vi "Load SA Parametersvi.vi"(8 "error in (no error)":errorcluster, 11 "Skyworks Spur Test in":refnum<class "Skyworks Spur Test.lvclass">) -> (0 "error out":errorcluster, 3 "Skyworks Spur Test out":refnum<class "Skyworks Spur Test.lvclass">)   [LabVIEW 2018, in "Skyworks Spur Test.lvlib" / "Skyworks Spur Test.lvclass"]
uses:
  Skyworks Spur Test.lvclass
  C:/Sequence Automation/Plugins/Measurement Interface.lvlibp/Measurement Interface.lvclass
  Controls/SA Parameters.ctl
  Skyworks Spur Test.lvclass/Skyworks Spur Test.ctl
  Write SA Parameters.vi
  Plugins/Measurement Interface.lvlibp/Private Methods/Measurement Parameters/Read Measurement Parameters.vi
  Plugins/String Database.lvlibp/String Database.lvclass
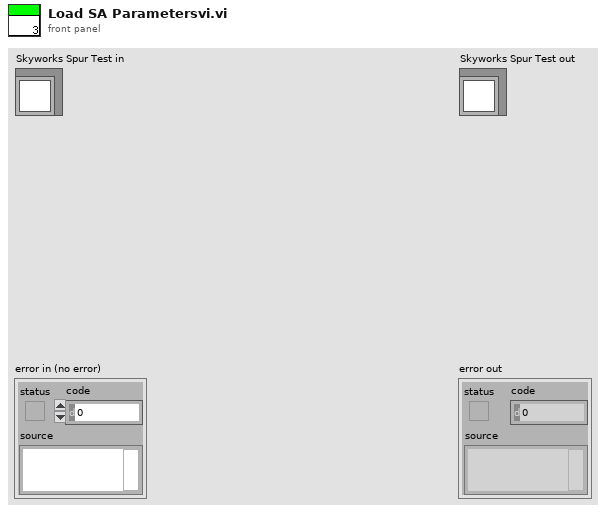
[diagram p1: front panel]
types:
  T1 = typedef "Skyworks Spur Test.lvlib/Skyworks Spur Test.lvclass/SA Parameters.ctl" = cluster{"Start Frequency":dbl, "Stop Frequency":dbl, "Bandwidth":dbl}
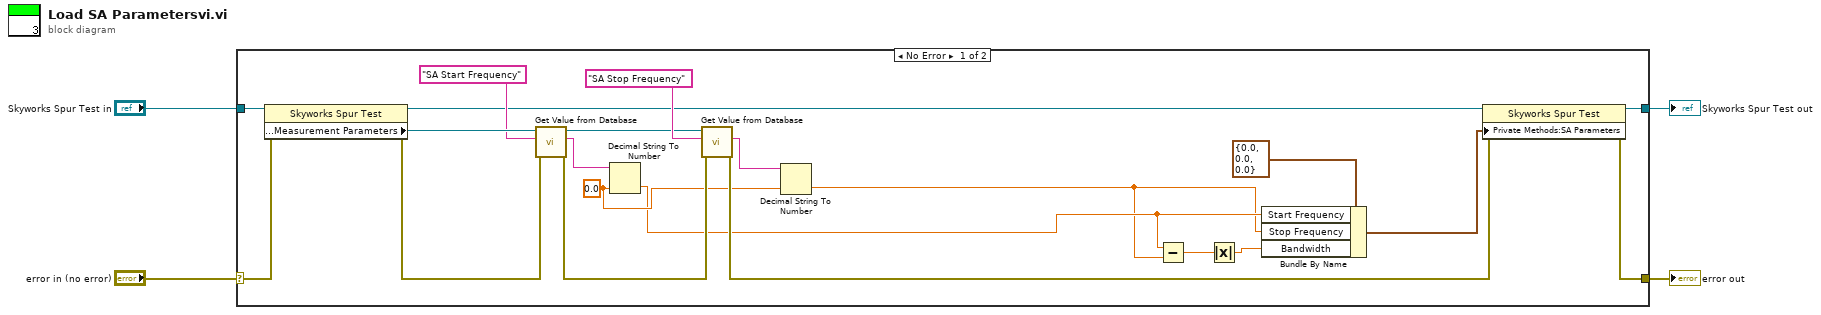
[diagram p0: block diagram]
diagram:
  n1 = case shown="No Error" "error in (no error)" {
    selector: "error in (no error)" -> [w25 w27]
    tunnel: [w18 w27] -> w3
    tunnel: [w16 w26] -> w1
    tunnel: "Skyworks Spur Test in" -> [w24 w26]
    frame No Error {
      w9 = 0.0 ("default (0 I32)")
      n2 = property class="Skyworks Spur Test"(reference=w24, error in=w25) -> (reference out=w17:refnum<class "Skyworks Spur Test.lvclass">, error out=w22:errorcluster, "Protected Methods:Measurement Parameters"=w23:refnum<class "String Database.lvclass">)
      n3 = call "Get Value from Database.vi"("error in (no error)"=w22, "Entry Name"="SA Start Frequency", "Message in"=w23) -> ("error out"=w12:errorcluster, "Entry Value"=w13:string, "Message out"=w19:refnum<class "String Database.lvclass">)  [unwired: 5 in, 1 out]
      n4 = Decimal String To Number(string=w13, default (0L)=w9) -> (number=w7:dbl)  [unwired: 1 in, 1 out]
      n5 = call "Get Value from Database.vi"("error in (no error)"=w12, "Entry Name"="SA Stop Frequency", "Message in"=w19) -> ("error out"=w11:errorcluster, "Entry Value"=w10:string)  [unwired: 5 in, 2 out]
      n6 = Decimal String To Number(string=w10, default (0L)=w9) -> (number=w6:dbl)  [unwired: 1 in, 1 out]
      n7 = Subtract(x=w7, y=w6) -> (x-y=w8:dbl)
      n8 = Absolute Value(x=w8) -> (abs(x)=w5:dbl)
      n9 = Bundle By Name(cluster=T1 {"Start Frequency"=0.0, "Stop Frequency"=0.0, "Bandwidth"=0.0} ("SA Parameters"), "Start Frequency"=w7, "Stop Frequency"=w6, "Bandwidth"=w5) -> (w14:T1)
      n10 = property class="Skyworks Spur Test"(reference=w17, error in=w11, "Private Methods:SA Parameters"=w14) -> (reference out=w16:refnum<class "Skyworks Spur Test.lvclass">, error out=w18:errorcluster)
    }
    frame Error {
    }
  }
  "error out" <- w3
  "Skyworks Spur Test out" <- w1
